vi "onConfigurePeeling.vi"(8 "error in (no error)":errorcluster, 11 "TraceabilityMatrix in":refnum<class "TraceabilityMatrix.lvclass">) -> (0 "error out":errorcluster, 3 "TraceabilityMatrix out":refnum<class "TraceabilityMatrix.lvclass">)   [LabVIEW 2021, in "Bananas.lvlib" / "TraceabilityMatrix.lvclass"]
uses:
  TraceabilityMatrix.lvclass
  TraceabilityMatrix.lvclass/TraceabilityMatrix.ctl
  <vilib>/LabVIEW Open Source Project/OpenURI/uri/URI.lvclass/URI.ctl
  9c1e9746-b5f7-48cc-898c-c7a44f4ab075.vi
  <vilib>/LabVIEW Open Source Project/OpenURI/components/path/Get path (absolute).vi
  <vilib>/LabVIEW Open Source Project/OpenURI/uri/URI.lvclass
  <vilib>/LabVIEW Open Source Project/OpenURI/openURI.lvlib
  Platano/Platano.lvclass
  <vilib>/LAVA/Robust CSV/Robust CSV.lvlib
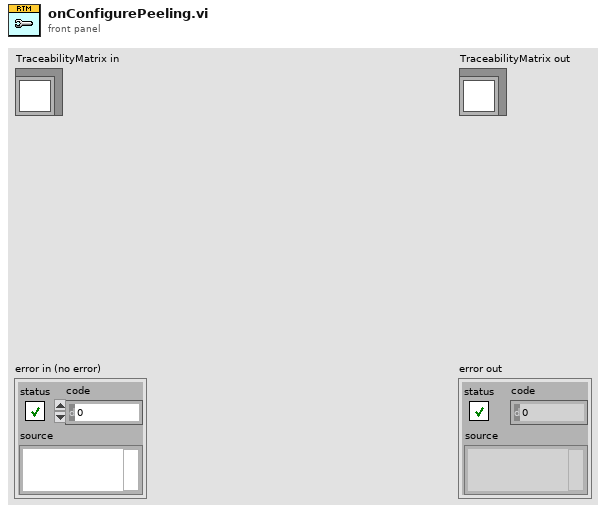
[diagram p1: front panel]
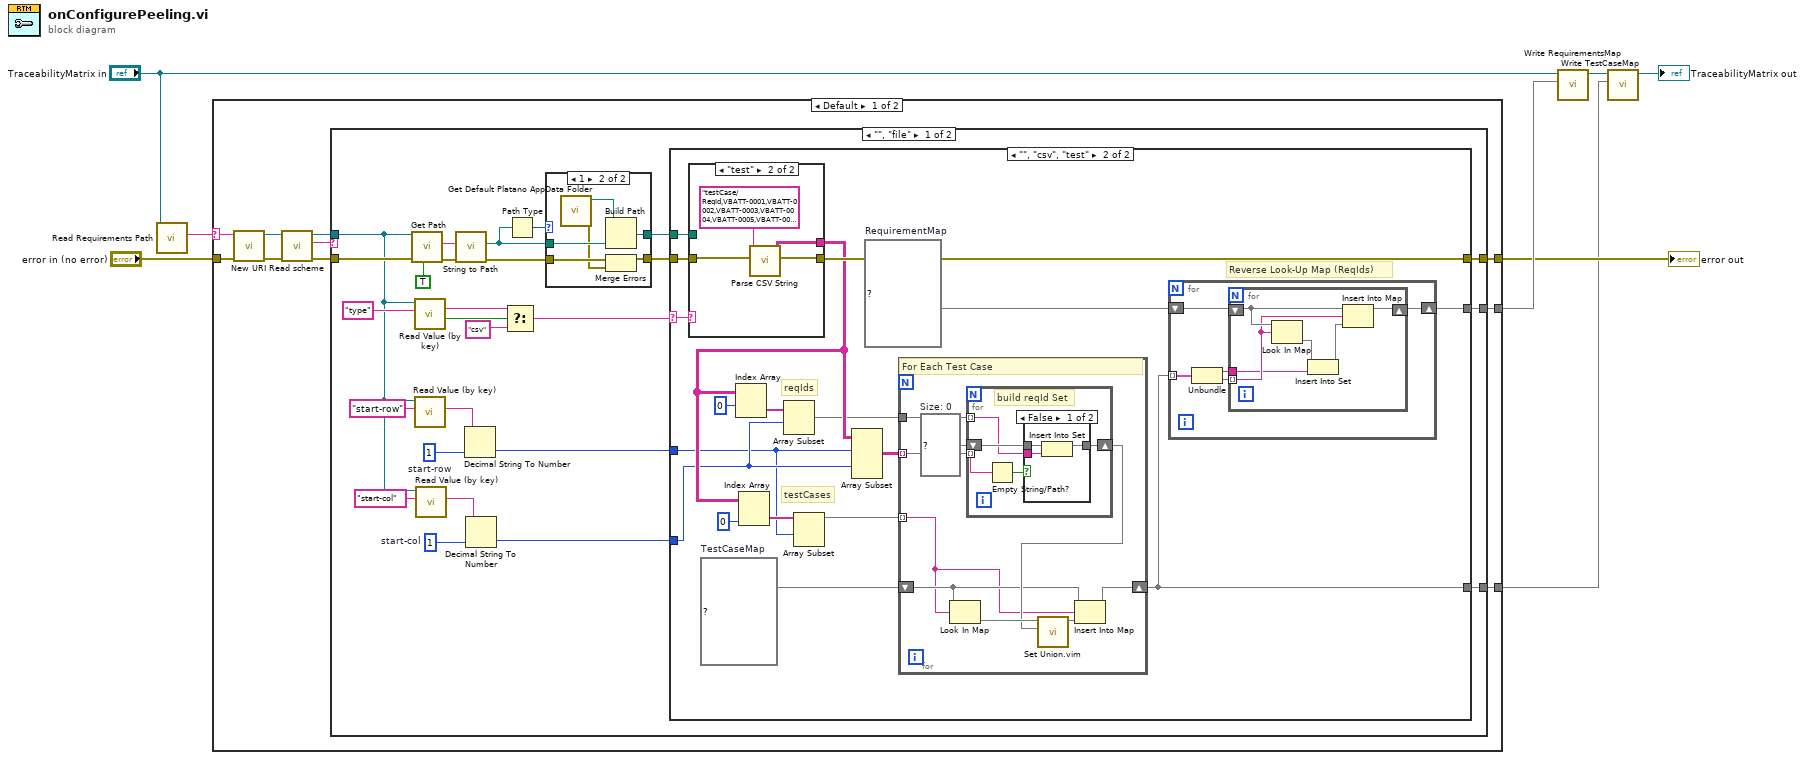
[diagram p0: block diagram]
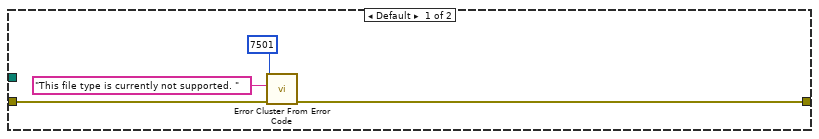
[diagram p2: hidden frame]
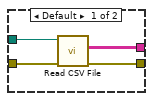
[diagram p4: hidden frame]
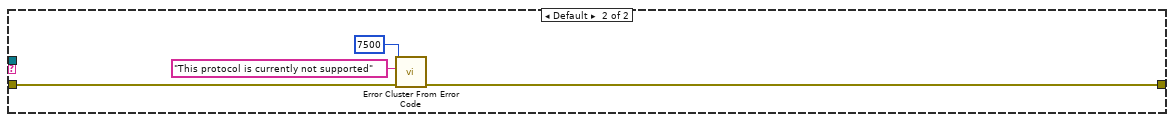
[diagram p6: hidden frame]
diagram:
  n1 = call "Read Requirements Path.vi"("Project in"="TraceabilityMatrix in") -> ("URI"=w6:string)  [unwired: 9 in, 1 out]
  n2 = case shown="Default" w6 {
    selector: w6 -> [w18 _]
    tunnel: [w10 _] -> w8
    tunnel: "error in (no error)" -> [w14 w115]
    tunnel: [w11 w115] -> w4
    tunnel: [w9 _] -> w1
    frame Default {
      n3 = call <vilib>:"New URI.vi"("error in (no error)"=w14, "URI"=w18) -> ("error out"=w13:errorcluster, "URI"=w15:refnum<class "URI.lvclass">)  [unwired: 8 in]
      n4 = call <vilib>:"Read scheme.vi"("error in (no error)"=w13, "URI in"=w15) -> ("error out"=w12:errorcluster, "scheme"=w16:string, "URI out"=w17:refnum<class "URI.lvclass">)  [unwired: 7 in]
      n5 = case shown="\"\", \"file\"" w16 {
        tunnel: w17 -> [w21 _]
        tunnel: w12 -> [w39 w113]
        tunnel: [w31 w114] -> w11
        tunnel: [w29 _] -> w10
        tunnel: [w19 _] -> w9
        frame "", "file" {
          w24 = 1  # start-col
          w26 = 1  # start-row
          n6 = call <vilib>:"Get Path.vi"("Strip lead \"/\" (F)"=TRUE ("Strip lead \"/\" (F)"), "error in (no error)"=w39, "URI in"=w21) -> ("error out"=w38:errorcluster, "path"=w42:string)  [unwired: 6 in, 1 out]
          n7 = call <vilib>:"Read Value (by key).vi"("key"="type", "URI in"=w21) -> ("found"=w36:bool, "value"=w35:string)  [unwired: 6 in, 2 out]
          n8 = call <vilib>:"Read Value (by key).vi"("key"="start-row", "URI in"=w21) -> ("value"=w27:string)  [unwired: 6 in, 3 out]
          n9 = call <vilib>:"Read Value (by key).vi"("key"="start-col", "URI in"=w21) -> ("value"=w23:string)  [unwired: 6 in, 3 out]
          n10 = call <vilib>:"String to Path.vi"("common path"=w42) -> ("Path"=w41:path)  [unwired: 10 in]
          n11 = Decimal String To Number(string=w27, default (0L)=w26) -> (number=w25:i32)  [unwired: 1 in, 1 out]
          n12 = Decimal String To Number(string=w23, default (0L)=w24) -> (number=w20:i32)  [unwired: 1 in, 1 out]
          n13 = Select(t=w35, s=w36, f="csv" ("key")) -> (s? t:f=w30:string)
          n14 = Path Type(1:w41) -> (0:w40:i16)
          n15 = case shown="1" w40 {
            tunnel: w41 -> [w104 w110]
            tunnel: [w104 w109] -> w33
            tunnel: w38 -> [w103 w108]
            tunnel: [w103 w106] -> w32
            frame Default {
            }
            frame 1 {
              n16 = call "Get Default Platano AppData Folder.vi"() -> ("error out"=w107:errorcluster, "Platano AppData"=w105:path)  [unwired: 10 in]
              n17 = Build Path(base path=w105, name or relative path=w110) -> (appended path=w109:path)
              n18 = Merge Errors(w108, w107) -> (w106:errorcluster)
            }
          }
          n19 = case shown="\"\", \"csv\", \"test\"" w30 {
            selector: w30 -> [_ w65]
            tunnel: w33 -> [_ w63]
            tunnel: w32 -> [w45 w64]
            tunnel: [w44 w62] -> w31
            tunnel: [_ w50] -> w29
            tunnel: w25 -> [_ w48]
            tunnel: w20 -> [_ w49]
            tunnel: [_ w52] -> w19
            frame Default {
              n20 = call <vilib>:"Error Cluster From Error Code.vi"("error in (no error)"=w45, "error message (\"\")"="This file type is currently not supported. " ("error message (\"\")"), "error code (0)"=7501) -> ("error out"=w44:errorcluster)  [unwired: 6 in]
            }
            frame "", "csv", "test" {
              w60 = map{string, set{string}} {}  # TestCaseMap
              w51 = map{string, set{string}} {}  # RequirementMap
              # "Reverse Look-Up Map (ReqIds)"
              # "testCases"
              # "reqIds"
              n21 = case shown="\"test\"" w65 {
                tunnel: w64 -> [w98 w101]
                tunnel: w63 -> [w97 _]
                tunnel: [w96 w100] -> w58
                tunnel: [w95 w102] -> w62
                frame Default {
                  n22 = call <vilib>:"Read CSV File.vi"("error in (no error)"=w98, "file path in"=w97) -> ("error out"=w95:errorcluster, "2-D array"=w96:string[][])  [unwired: 7 in, 1 out]
                }
                frame "test" {
                  n23 = call <vilib>:"Parse CSV String.vi"("error in"=w101, "CSV string"="testCase/ReqId,VBATT-0001,VBATT-0002,VBATT-0003,VBATT-0004,VBATT-0005,VBATT-0006\nBatteryVoltage - LOW,x,,,,,\nBatteryVoltage - NOMINAL,,,x,,,x\nBatteryVoltage - HIGH,,,,x,x,\nBatteryVoltage - SHORT,,x,,,,\nBatteryVoltage - REVERSE,x,x,,,,") -> ("error out"=w102:errorcluster, "2-D array"=w100:string[][])  [unwired: 3 in, 5 out]
                }
              }
              n24 = Index Array(array=w58, index (row)=0) -> (element=w56:string[])  [unwired: 1 in]
              n25 = Index Array(array=w58, index (col)=0 ("index (row)")) -> (element=w54:string[])  [unwired: 1 in]
              n26 = Array Subset(array=w56, index=w49) -> (w55:string[])  [unwired: 1 in]
              n27 = Array Subset(array=w54, index=w48) -> (w53:string[])  [unwired: 1 in]
              n28 = Array Subset(array=w58, index (row)=w48, index (col)=w49) -> (w61:string[][])  [unwired: 2 in]
              n29 = for {
                tunnel: w61 -> [w85] mode=indexing
                shift-right: [w78] -> w52
                shift-left: w60 -> [w79]
                tunnel: w53 -> [w77] mode=indexing
                tunnel: w55 -> [w83]
                w84 = set{string} {}  # Size: 0
                # "For Each Test Case"
                n30 = Look In Map(map=w79, key=w77) -> (value=w82:set{string})  [unwired: 1 in, 1 out]
                n31 = for {
                  tunnel: w85 -> [w88] mode=indexing
                  shift-right: [w90] -> w81
                  shift-left: w84 -> [w89]
                  tunnel: w83 -> [w86] mode=indexing
                  # "build reqId Set"
                  n32 = Empty String/Path?(string/path=w88) -> (empty?=w87:bool)
                  n33 = case shown="False" w87 {
                    tunnel: [w93 w94] -> w90
                    tunnel: w89 -> [w92 w94]
                    tunnel: w86 -> [w91 _]
                    frame False {
                      n34 = Insert Into Set(10:w91, 11:w92) -> (3:w93:set{string})  [unwired: 1 out]
                    }
                    frame True {
                    }
                  }
                }
                n35 = call "Set Union.vim"("set 2"=w81, "set 1"=w82) -> ("union"=w80:set{string})  [unwired: 9 in]
                n36 = Insert Into Map(map in=w79, key=w77, value=w80) -> (map out=w78:map{string, set{string}})  [unwired: 2 out]
              }
              n37 = for {
                tunnel: w52 -> [w70] mode=indexing
                shift-right: [w68] -> w50
                shift-left: w51 -> [w69]
                n38 = Unbundle(w70) -> ("testCase"=w66:string, "reqIds"=w67:set{string})
                n39 = for {
                  tunnel: w67 -> [w74] mode=indexing
                  tunnel: w66 -> [w71]
                  shift-right: [w75] -> w68
                  shift-left: w69 -> [w76]
                  n40 = Look In Map(map=w76, key=w74) -> (value=w73:set{string})  [unwired: 1 in, 1 out]
                  n41 = Insert Into Set(10:w71, 11:w73) -> (3:w72:set{string})  [unwired: 1 out]
                  n42 = Insert Into Map(map in=w76, key=w74, value=w72) -> (map out=w75:map{string, set{string}})  [unwired: 2 out]
                }
              }
            }
          }
        }
        frame Default {
          n43 = call <vilib>:"Error Cluster From Error Code.vi"("error in (no error)"=w113, "error message (\"\")"="This protocol is currently not supported" ("error message (\"\")"), "error code (0)"=7500) -> ("error out"=w114:errorcluster)  [unwired: 6 in]
        }
      }
    }
    frame "" {
    }
  }
  "error out" <- w4
  n44 = call "Write RequirementsMap.vi"("RequirementMap"=w8, "RequirementsFile in"="TraceabilityMatrix in") -> ("RequirementsFile out"=w3:refnum<class "TraceabilityMatrix.lvclass">)  [unwired: 9 in]
  n45 = call "Write TestCaseMap.vi"("TestCaseMap"=w1, "RequirementsFile in"=w3) -> ("RequirementsFile out"=→"TraceabilityMatrix out":refnum<class "TraceabilityMatrix.lvclass">)  [unwired: 9 in]
